vi "debug_randled.vi"() -> ()   [LabVIEW 2012]
uses:
  <vilib>/Platform/TimedLoop/XDataNode/XDataNode.xnode
  <vilib>/Platform/TimedLoop/XDataNode/nitl_modes.ctl
  <vilib>/Platform/TimedLoop/XDataNode/XDNodeRunTimeDep.lvlib
  <vilib>/Platform/TimedLoop/XDataNode/wakeup.ctl
  <vilib>/Platform/TimedLoop/XDataNode/timing_clust.ctl
panel:
  out "Turnaround counter":u32
  out "Error!":bool
  out "Total number of times is test pulse has blinked":i16
  out "Testpulse Separation (20 ns ticks)":u32=500
  out "Test pulse address":i16
  in  "stop":bool
  out "State?":bool
  out "Test Pulse Counter":u32
  out "Total number of pulses sent":u64
  in  "Testpulse Time Delay (20 ns ticks)":u32=15
  in  "Testpulse duration (20 ns ticks)":u32=1
  in  "FPGA I/O In":refnum<k21>="IO Module\\D0 0"
  out "Is Test Pulse?":bool
  in  "Testpulser On/Off":bool
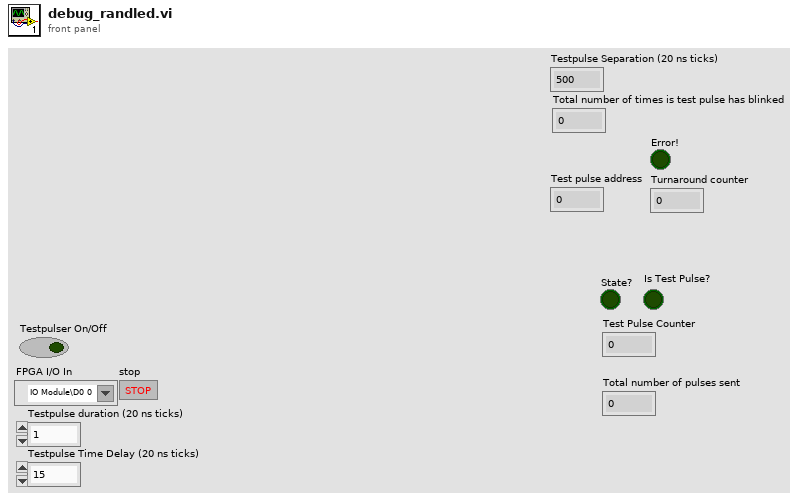
[diagram p1: front panel]
types:
  T1 = typedef "XDNodeRunTimeDep.lvlib/timing_clust.ctl" = cluster{"Expected End [f-1]":u64, "Actual End [f-1]":u64, "Finished Late? [f-1]":bool, "Expected End [i-1]":u64, "Actual End [i-1]":u64, "Finished Late? [i-1]":bool, "Expected Start [i]":u64, "Actual Start [i]":u64, "Expected Start [f]":u64, "Actual Start [f]":u64, "Source Name":string, "Structure Name":string, "Period":i64, "Deadline":i64, "Offset":i64, "Start":i64, "Priority":i32, "Timeout":i32, "Mode":T2, "Wakeup Reason":T3, "Error":errorcluster, "Source Type":string, "Secondary Source Type":string, "Global End Time":u64, "Global Start Time":u64, "Frame Duration":u64, "Iteration Duration":u64, "Assigned CPU":i32, "I/O Scan Engine Mode":u32}
  T2 = typedef "XDNodeRunTimeDep.lvlib/nitl_modes.ctl" = enum32{"No Change", "Process missed periods, maintain original phase", "Discard missed periods, maintain original phase", "Process missed periods, ignore original phase", "Discard missed periods, ignore original phase"}
  T3 = typedef "XDNodeRunTimeDep.lvlib/wakeup.ctl" = enum32{"Normal", "Aborted", "Asynchronous wakeup", "Timing source error", "Timed loop error", "Timeout"}
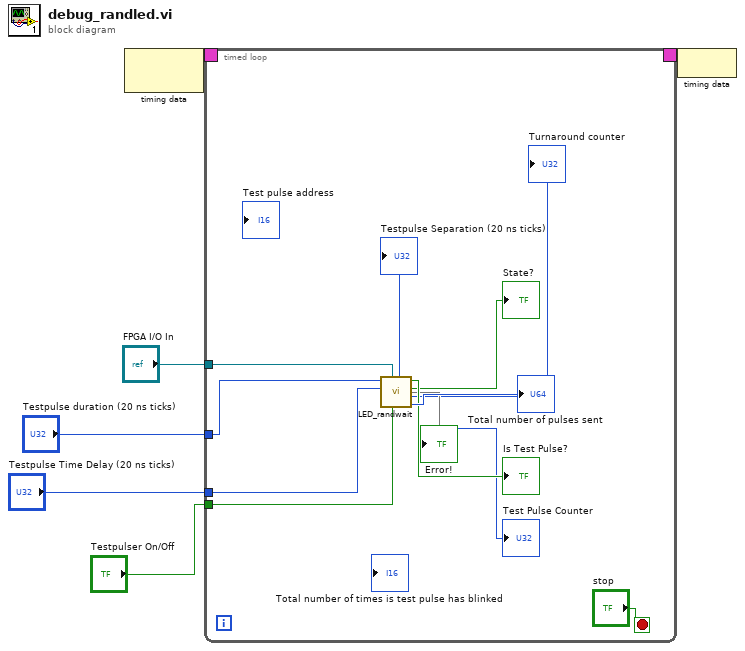
[diagram p0: block diagram]
diagram:
  n1 = node-c288() -> (w2:T1)  [unwired: 1 in]
  n2 = timed-loop {
    tunnel: "Testpulser On/Off" -> [w9]
    tunnel: "FPGA I/O In" -> [w14]
    tunnel: "Testpulse duration (20 ns ticks)" -> [w16]
    tunnel: "Testpulse Time Delay (20 ns ticks)" -> [w15]
    timing: w2 -> [_]
    timing-out: [_] -> w1
    stop <- "stop" stop-if-true
    n3 = call "LED_randwait.vi"("Testpulser On/Off 2"=w9, "FPGA I/O In 2"=w14, "Testpulse Time Delay (20 ns ticks) 2"=w15, "Testpulse duration (20 ns ticks) 2"=w16) -> ("Total number of pulses sent 2"=→"Total number of pulses sent":u64, "Counter"=→"Test Pulse Counter":u32, "State? 2"=→"State?":bool, "Is Test Pulse? 2"=→"Is Test Pulse?":bool, 4:→"Error!", "Test Pulse separation"=→"Testpulse Separation (20 ns ticks)":u32, "Turnaround counter"=→"Turnaround counter":u32)  [unwired: 1 in]
  }
  n4 = node-c288(w1) -> ()
